vi "Deploy Libraries.vi"(8 "Error In":errorcluster, 10 "Library Paths":path[](array[path]), 11 "CS++DSCManager in":refnum<class "CS++DSCManager.lvclass">) -> (0 "Error Out":errorcluster, 3 "CS++DSCManager out":refnum<class "CS++DSCManager.lvclass">)   [LabVIEW 2014, in "CS++DSCManager.lvlib" / "CS++DSCManager.lvclass"]
doc: "Deploys the variables in multiple LabVIEW project libraries into the Shared Variable Engine (SVE) on the host computer. The variables are in a running state. This operation is available only on the host computer, so any VIs contained in the project libraries remain unaffected."
uses:
  CS++DSCManager.lvclass
  <vilib>/lvdsc/process/internal/PRC_DeployLibraries.vi
  <vilib>/lvdsc/NI_DSC.lvlib
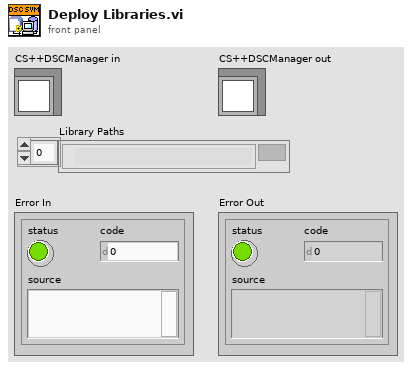
[diagram p1: front panel]
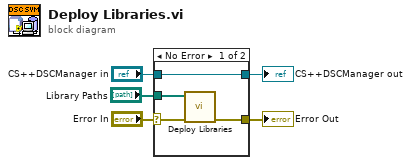
[diagram p0: block diagram]
diagram:
  n1 = case shown="No Error" "Error In" {
    selector: "Error In" -> [w9 w11]
    tunnel: [w7 w11] -> w4
    tunnel: [w8 w10] -> w2
    tunnel: "CS++DSCManager in" -> [w8 w10]
    tunnel: "Library Paths" -> [w6 _]
    frame No Error {
      n2 = call-poly <vilib>:"Deploy Libraries.vi"("error in (no error)"=w9, "library paths"=w6) -> ("error out"=w7:errorcluster)  [unwired: 7 in]
    }
    frame Error {
    }
  }
  "Error Out" <- w4
  "CS++DSCManager out" <- w2
